vi "Temperature Monitor.vi"() -> ()   [LabVIEW 2025]
doc: "This VI is the solution to an exercise in the LabVIEW Core 1 course.\n\nIt uses a While Loop and shift registers to average data. No hardware is necessary."
panel:
  out "deleted portion":dbl[][](array[numeric])
  out "array w/ subset deleted":dbl[][](array[numeric])
  in  "index (row)":i32
  in  "length":i32
  out "output array":i32[][](array[numeric])
  in  "Stop Button":bool
  out "Temperature History":cluster{dbl, "Temperature Value":dbl}(graph)
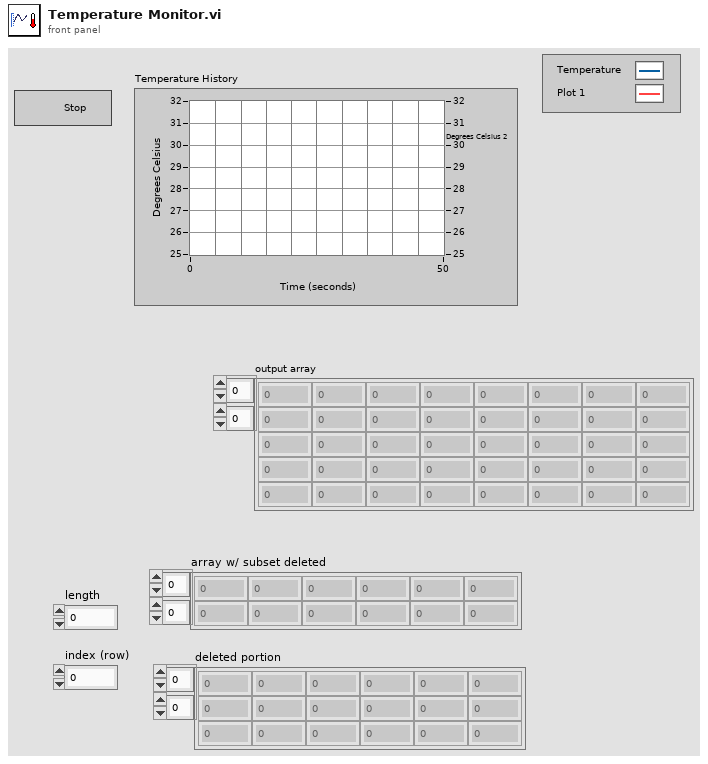
[diagram p1: front panel]
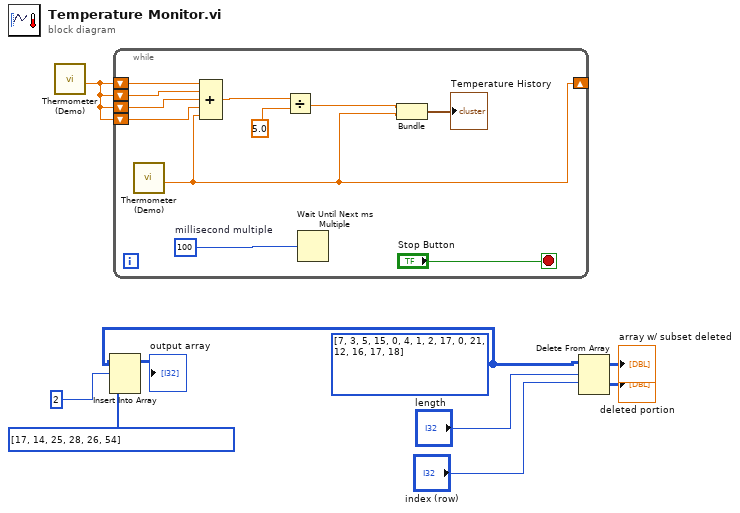
[diagram p0: block diagram]
diagram:
  w2 = i32[][] [[7, 3, 5, 15, 0], [4, 1, 2, 17, 0], [21, 12, 16, 17, 18]] ("array")
  n1 = call "Thermometer (Demo).vi"() -> ("Temperature Value"=w9:dbl)  [unwired: 11 in]
  n2 = Insert Into Array(array=w2, index (row)=2, new element=i32[] [17, 14, 25, 28, 26, 54] ("new element/subarray")) -> (→"output array":i32[][])  [unwired: 1 in]
  n3 = while {
    shift-right: [w10] -> _
    shift-left: w9 -> [w18]
    shift-left: w9 -> [w17]
    shift-left: w9 -> [w16]
    shift-left: w9 -> [w13]
    stop <- "Stop Button" stop-if-true
    w20 = u32 100  # millisecond multiple
    n4 = call "Thermometer (Demo).vi"() -> ("Temperature Value"=w10:dbl)  [unwired: 11 in]
    n5 = Compound Arithmetic op=ADD(w18, w17, w16, w13, w10) -> (w15:dbl)
    n6 = Divide(x=w15, y=5.0) -> (x/y=w11:dbl)
    n7 = Wait Until Next ms Multiple(millisecond multiple=w20) -> ()  [unwired: 1 out]
    n8 = Bundle(w11, "Temperature Value"=w10) -> (→"Temperature History":cluster{dbl, "Temperature Value":dbl})  [unwired: 1 in]
  }
  n9 = Delete From Array(array=w2, length="length", index (row)="index (row)") -> (deleted portion=→"deleted portion":i32[][], array with subset deleted=→"array w/ subset deleted":i32[][])  [unwired: 1 in]
